vi "timeout.vi"(8 "error in (no error)":errorcluster, 9 "timeout_secs":u64, 10 "connect_timeout_secs":u64, 11 "ClientBuilder in":refnum<class "Headers.lvclass">) -> (0 "error out":errorcluster, 3 "ClientBuilder out":refnum<class "Headers.lvclass">)   [LabVIEW 2020, in "reqwest.lvlib" / "Headers.lvclass"]
uses:
  Headers.lvclass
  Headers.lvclass/Headers.ctl
  lv_reqwest_64.dll
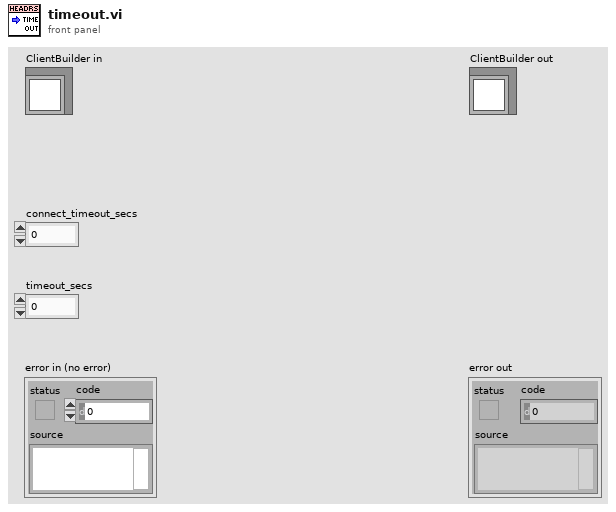
[diagram p1: front panel]
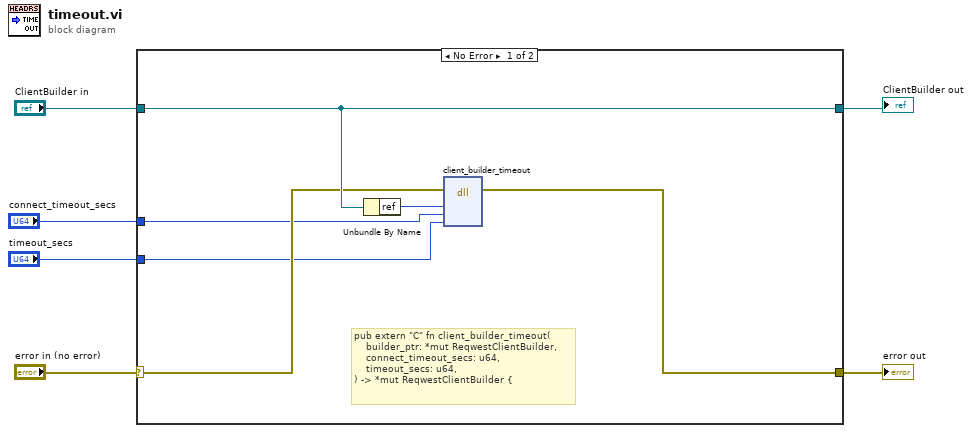
[diagram p0: block diagram]
diagram:
  n1 = case shown="No Error" "error in (no error)" {
    selector: "error in (no error)" -> [w9 w13]
    tunnel: "ClientBuilder in" -> [w10 w14]
    tunnel: [w12 w13] -> w3
    tunnel: [w10 w14] -> w4
    tunnel: "connect_timeout_secs" -> [w8 _]
    tunnel: "timeout_secs" -> [w7 _]
    frame No Error {
      # "pub extern \"C\" fn client_builder_timeout(\n    builder_ptr: *mut ReqwestClientBuilder,\n    connect_timeout_secs: u64,\n    timeout_secs: u64,\n) -> *mut ReqwestClientBuilder {"
      n2 = Unbundle By Name(w10) -> ("ref"=w11:u64)
      n3 = dll-call lib="C:/Projects/reqwest-rs-labview/lv_src/lv_reqwest_64.dll" fn="client_builder_timeout"(error in=w9, "client_builder_ref"=w11, "connect_timeout_secs"=w8, "timeout_secs"=w7) -> (error out=w12:errorcluster)  [unwired: 6 in, 1 out]
    }
    frame Error {
    }
  }
  "error out" <- w3
  "ClientBuilder out" <- w4
